vi "PGPASS.dialog.vi"(8 "error in (no error)":errorcluster) -> (0 "error out":errorcluster, 3 "Connection Information":T1)   [LabVIEW 2019, in "PGPASS.lvlib"]
uses:
  PGPASS.lvlib
  PGPASS.Connection Information.ctl
panel:
  in  "OK":bool
  in  "hostname":string
  in  "port":string
  in  "dbname":string
  in  "user":string
  in  "password":string
  # "Connection not found.\nPlease enter info below."
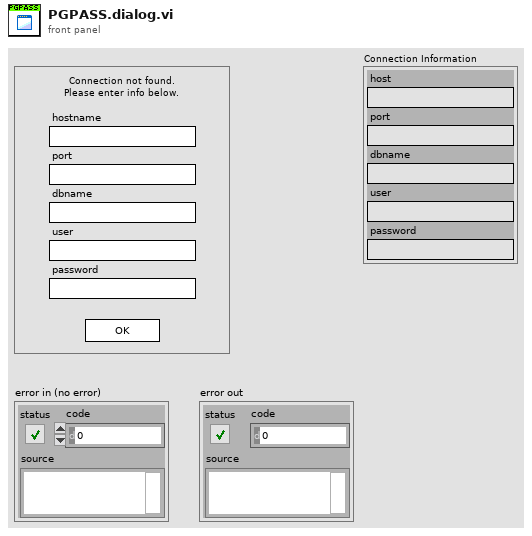
[diagram p1: front panel]
types:
  T1 = typedef "PGPASS.lvlib/PGPASS.Connection Information.ctl" = cluster{"host":string, "port":string, "dbname":string, "user":string, "password":string}
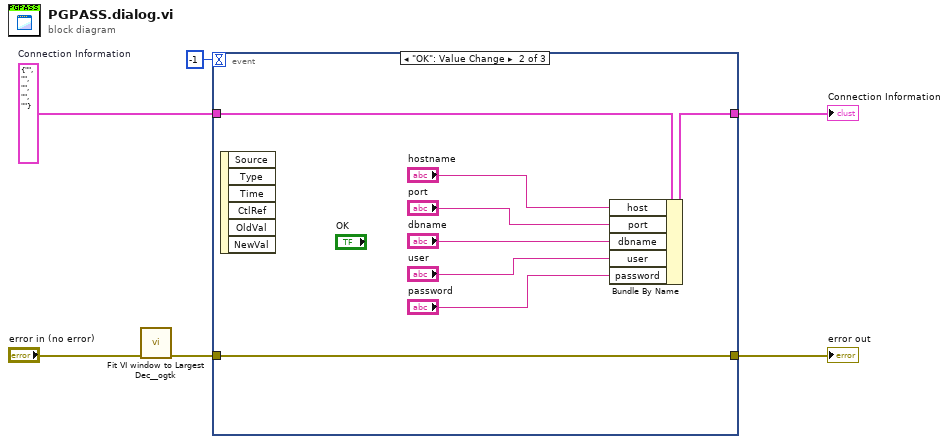
[diagram p0: block diagram]
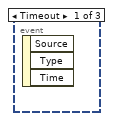
[diagram p2: hidden frame]
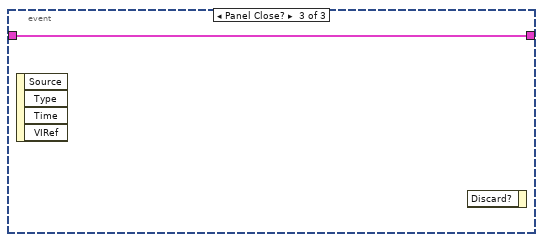
[diagram p3: hidden frame]
diagram:
  w5 = T1 {"host"="", "port"="", "dbname"="", "user"="", "password"=""}  # Connection Information
  n1 = call <userlib>:"Fit VI window to Largest Dec__ogtk.vi"("error in (no error)"="error in (no error)") -> ("error out"=w3:errorcluster)  [unwired: 5 in, 1 out]
  n2 = event shown="[1] \"OK\": Value Change" {
    selector: _ -> [_ _ _]
    dyn-events: _ -> [_ _ _]
    timeout: -1 -> [_ _ _]
    tunnel: w5 -> [_ w14 w15]
    tunnel: [_ w8 w15] -> w4
    tunnel: w3 -> [_ w7 _]
    tunnel: [_ w7 _] -> w2
    event Timeout {
      n3 = event-data() -> ()  [unwired: 1 in, 3 out]
    }
    event "OK": Value Change {
      n4 = event-data() -> ()  [unwired: 1 in, 6 out]
      n5 = Bundle By Name(cluster=w14, "host"="hostname", "port"="port", "dbname"="dbname", "user"="user", "password"="password") -> (w8:T1)
    }
    event Panel Close? {
      n6 = event-data() -> ()  [unwired: 1 in, 4 out]
      n7 = event-data() -> ()  [unwired: 2 in, 1 out]
    }
  }
  "error out" <- w2
  "Connection Information" <- w4
